vi "ReadWrite.Initialize.vi"(8 "error in":errorcluster, 10 "VS Engine Interface":refnum<class "VS Engine Interface.lvclass">, 11 "Settings":T2 {"Refs" format="%.0x"}) -> (0 "error out":errorcluster, 3 "ReadWrite out":refnum<class "ReadWrite.lvclass">)   [LabVIEW 2024, in "VS Plugin Inline Async API.lvlib" / "ReadWrite.lvclass"]
uses:
  ReadWrite.lvclass
  ReadWrite.lvclass/ReadWrite.ctl
  <vilib>/NI VeriStand/Custom Device API/Data Reference.ctl
  <vilib>/NI VeriStand/Custom Device API/Custom Device API.lvlib
  VS Engine Abstraction/VS Engine Interface/VS Engine Interface.lvclass
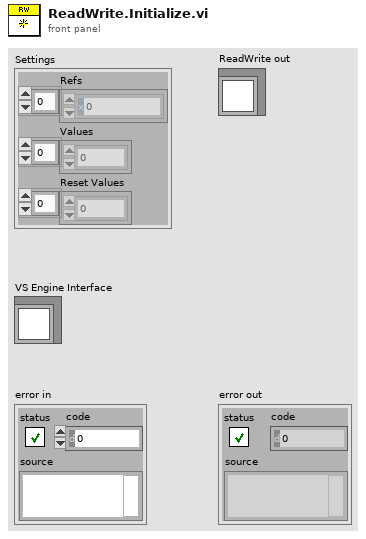
[diagram p1: front panel]
types:
  T1 = typedef "Custom Device API.lvlib/Data Reference.ctl" = i32
  T2 = cluster{"Refs":T1[], "Values":dbl[], "Reset Values":dbl[]}
  T3 = cluster{"read mode":enum16{"polling", "blocking"}, "write mode":enum16{"polling", "blocking"}}
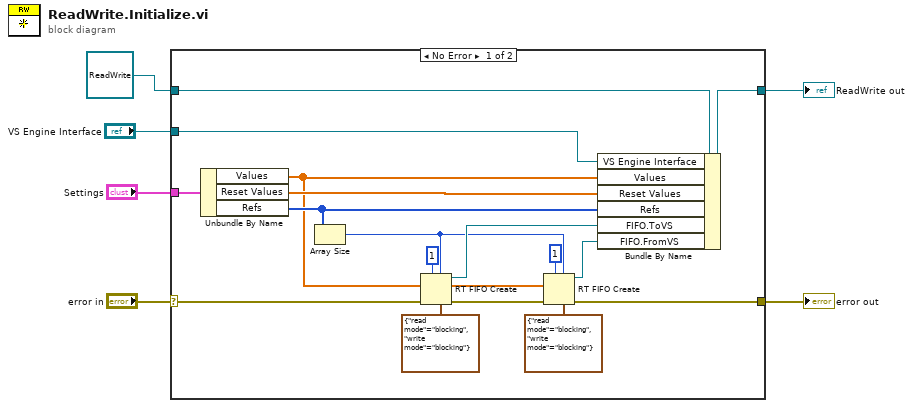
[diagram p0: block diagram]
diagram:
  n1 = case shown="No Error" "error in" {
    selector: "error in" -> [w21 w25]
    tunnel: [w23 w25] -> w5
    tunnel: refnum<class "ReadWrite.lvclass"> refnum ("ReadWrite in") -> [w13 w24]
    tunnel: [w12 w24] -> w2
    tunnel: "Settings" -> [w11 _]
    tunnel: "VS Engine Interface" -> [w7 _]
    frame No Error {
      n2 = Unbundle By Name(w11) -> ("Values"=w8:dbl[], "Reset Values"=w9:dbl[], "Refs"=w10:T1[])
      n3 = Array Size(array=w10) -> (size(s)=w14:i32)
      n4 = RT FIFO Create(1:w8, 3:w21, 4:u32 1 ("size (10)"), 6:w14, 7:T3 {"read mode"=enum."blocking", "write mode"=enum."blocking"} ("r/w modes (polling,polling)")) -> (8:w19:refnum<k33>, 11:w22:errorcluster)  [unwired: 3 in, 1 out]
      n5 = RT FIFO Create(1:w8, 3:w22, 4:u32 1 ("size (10)"), 6:w14, 7:T3 {"read mode"=enum."blocking", "write mode"=enum."blocking"} ("r/w modes (polling,polling)")) -> (8:w20:refnum<k33>, 11:w23:errorcluster)  [unwired: 3 in, 1 out]
      n6 = Bundle By Name(cluster=w13, "VS Engine Interface"=w7, "Values"=w8, "Reset Values"=w9, "Refs"=w10, "FIFO.ToVS"=w19, "FIFO.FromVS"=w20) -> (w12:refnum<class "ReadWrite.lvclass">)
    }
    frame Error {
    }
  }
  "error out" <- w5
  "ReadWrite out" <- w2
